vi "LAT_Long Dist.vi"(8 "long_DTU":dbl, 9 "long":dbl, 10 "lat_DTU":dbl format="%#_6f", 11 "lat":dbl) -> (3 "Distance":dbl format="%#_6f")   [LabVIEW 2024]
panel:
  out "a":dbl format="%#_6f"
  out "output variable":dbl format="%#_6f"
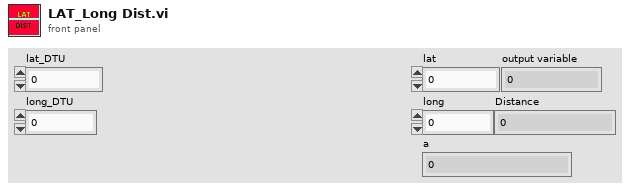
[diagram p1: front panel]
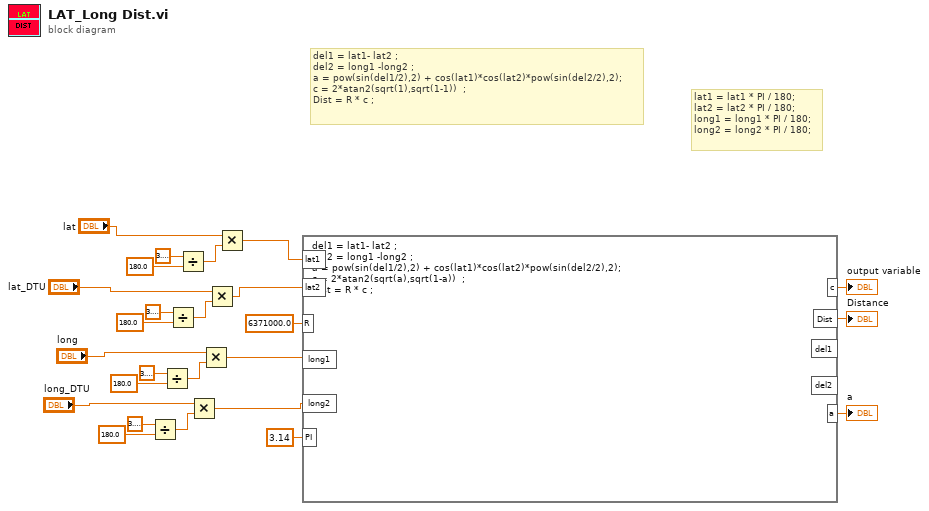
[diagram p0: block diagram]
diagram:
  # "del1 = lat1- lat2 ;\ndel2 = long1 -long2 ;\na = pow(sin(del1/2),2) + cos(lat1)*cos(lat2)*pow(sin(del2/2),2);\nc = 2*atan2(sqrt(1),sqrt(1-1))  ;\nDist = R * c ;"
  # "lat1 = lat1 * PI / 180;\nlat2 = lat2 * PI / 180;\nlong1 = long1 * PI / 180;\nlong2 = long2 * PI / 180;"
  n1 = Divide(x=3.141592653589793, y=180.0) -> (x/y=w4:dbl)
  n2 = Divide(x=3.141592653589793, y=180.0) -> (x/y=w9:dbl)
  n3 = Divide(x=3.141592653589793, y=180.0) -> (x/y=w14:dbl)
  n4 = Divide(x=3.141592653589793, y=180.0) -> (x/y=w18:dbl)
  n5 = Multiply(x="long_DTU", y=w4) -> (x*y=w2:dbl)
  n6 = Multiply(x="long", y=w9) -> (x*y=w7:dbl)
  n7 = Multiply(x="lat_DTU", y=w14) -> (x*y=w12:dbl)
  n8 = Multiply(x="lat", y=w18) -> (x*y=w17:dbl)
  n9 = formula code="del1 = lat1- lat2 ;\ndel2 = long1 -long2 ;\na = pow(sin(del1/2),2) + cos(lat1)*cos(lat2)*pow(sin(del2/2),2);\nc = 2*atan2(sqrt(a),sqrt(1-a))  ;\nDist = R * c ;"("R"=6371000.0 ("input variable"), "lat1"=w17, "lat2"=w12, "long1"=w7, "long2"=w2, "PI"=3.14 ("input variable")) -> ("c"=→"output variable":dbl, "Dist"=→"Distance":dbl, "a"=→"a":dbl)  [unwired: 2 out]
